vi "Get IVIControls Name.vi"(11 "error in (no error)":errorcluster) -> (4 "Control Names Out":string[](array[string]), 6 "Array Size":i32, 15 "error out":errorcluster)   [LabVIEW 2021, in "Migrator Reusables.lvlib"]
uses:
  Migrator Reusables.lvlib
  controls/Dictionary States.ctl
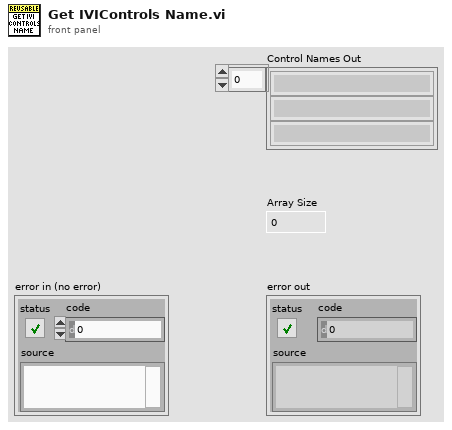
[diagram p1: front panel]
types:
  T1 = typedef "Migrator Reusables.lvlib/Dictionary States.ctl" = enum16{"Set", "Get", "Delete", "Delete All"}
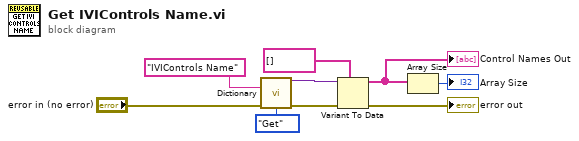
[diagram p0: block diagram]
diagram:
  n1 = call "Dictionary.vi"("Key"="IVIControls Name", "error in (no error)"="error in (no error)", "Dict States"=Dictionary_States."Get") -> ("Variant_Out"=w5:variant, "error out"=w6:errorcluster)  [unwired: 11 in]
  n2 = Variant To Data(error in=w6, type=string[] [], Variant=w5) -> (data=w2:string[], error out=→"error out":errorcluster)
  "Control Names Out" <- w2
  n3 = Array Size(array=w2) -> (size(s)=→"Array Size":i32)
